vi "TagDB Using regexp Example.vi"() -> ()   [LabVIEW 2017]
uses:
  4f433c9a-a00c-49f1-9e84-35b769afccce.vi
  8cf9f43b-58a1-407a-9b53-072bd7cbe5d9.vi
  TagDB/_Support/DataAccess/data-Write.vi
  TagDB/_Support/Error/_[error50000]Invalid DB REF.vi
  TagDB/_Support/DataAccess/TagDB Ref to DVR.vi
  TagDB/_Support/Change Detector/TagDB dbChanged.vi
  TagDB/_Support/Error/_Clear Errors.vi
  8cf9f43b-58a1-407a-9b53-072bd7cbe5d9.vi/29b2ea6d-6d7f-4e4a-ad31-a5cb760462c7.vi
  TagDB/API/TagDB-Status.vi
  TagDB/_Support/DataAccess/_NameCacher.vi
  TagDB/_Support/DataAccess/_datatypeChecker.vi
  TagDB/_Support/Change Detector/TagDB ChangeFlag.vi
  TagDB/_Support/Error/_[error50002]Invalid DataType.vi
  TagDB/_Support/URL/TRIM-BOTH-SPACE.vi
  <vilib>/Utility/Data Type/Get Type Information.vi
  TagDB/_Support/Error/_Build Error Cluster.vi
  TagDB/TagDB.lvlib
panel:
  out "names Sorted":string[](array[string])
  out "value":i32[][](array[numeric])
  out "names":string[](array[string])
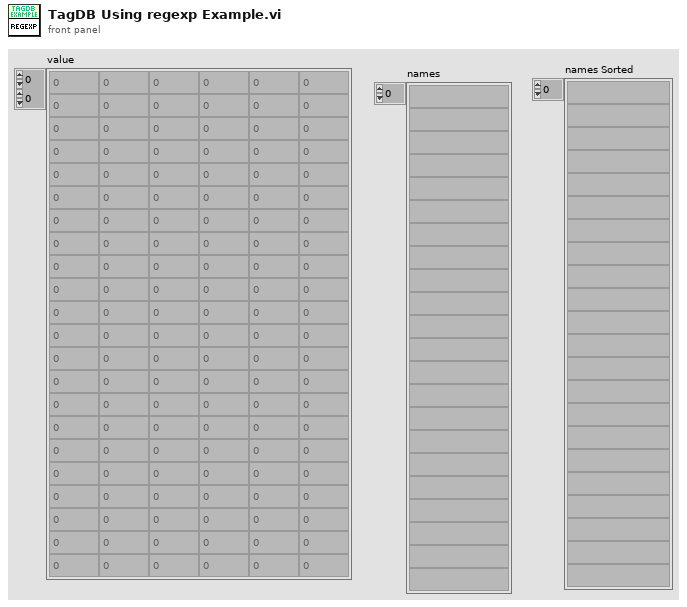
[diagram p1: front panel]
types:
  T1 = typedef "TagDB.lvlib/TagDB.ctl" = refnum<k1>
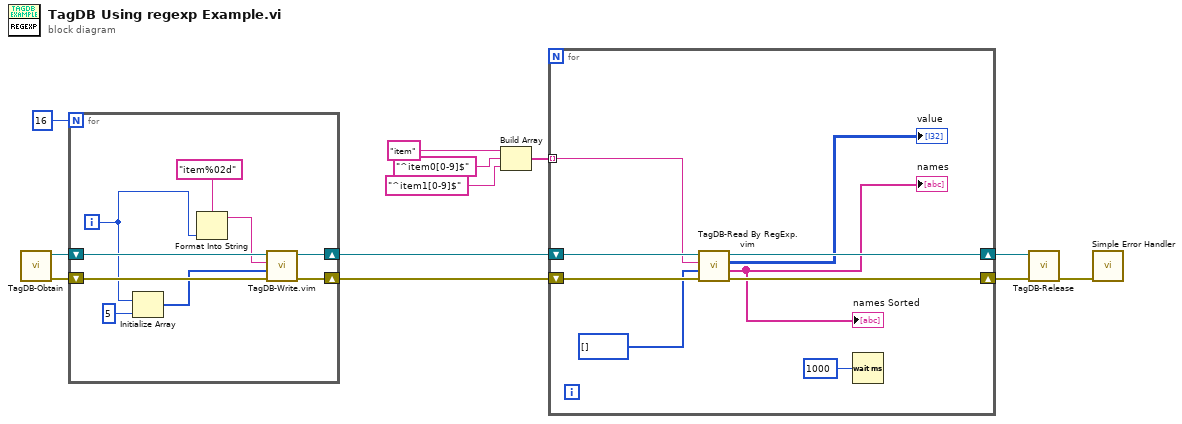
[diagram p0: block diagram]
diagram:
  n1 = call "TagDB-Obtain.vi"() -> ("error out"=w8:errorcluster, "TagDB"=w9:T1)  [unwired: 5 in, 1 out]
  n2 = for {
    N: 16 -> [_]
    shift-right: [w19] -> w11
    shift-left: w9 -> [w21]
    shift-right: [w18] -> w10
    shift-left: w8 -> [w20]
    i -> [w14]
    n3 = Initialize Array(w14, 5 ("dimension size")) -> (w15:i32[])
    n4 = Format Into String(format string="item%02d" ("String"), w14) -> (resulting string=w16:string)  [unwired: 2 in, 1 out]
    n5 = call "TagDB-Write.vim"("error in (no error)"=w20, "Value"=w15, "tag"=w16, "TagDB"=w21) -> ("error out"=w18:errorcluster, "TagDB(dup)"=w19:T1)  [unwired: 5 in, 1 out]
  }
  n6 = Build Array("item", "^item0[0-9]$", "^item1[0-9]$") -> (w3:string[])
  n7 = for {
    shift-right: [w30] -> w1
    shift-left: w11 -> [w28]
    shift-right: [w29] -> w12
    shift-left: w10 -> [w27]
    tunnel: w3 -> [w22] mode=indexing
    n8 = call "TagDB-Read By RegExp.vim"("error in (no error)"=w27, "Type"=i32[] [], "RegExp"=w22, "DB Ref"=w28) -> ("error out"=w29:errorcluster, "names"=→"names" →"names Sorted":string[], "value"=→"value":i32[][], "DB Ref(dup)"=w30:T1)  [unwired: 4 in]
    n9 = Wait (ms)(milliseconds to wait=u32 1000) -> ()  [unwired: 1 out]
  }
  n10 = call "TagDB-Release.vi"("error in (no error)"=w12, "TagDB"=w1) -> ("error out"=w2:errorcluster)  [unwired: 9 in]
  n11 = call <vilib>:"Simple Error Handler.vi"("error in (no error)"=w2) -> ()  [unwired: 4 in, 5 out]
